vi "CRYXY Graph InsDel.vi"(10 "Graph VI Ref":refnum<vi>, 11 "sAction":string) -> ()   [LabVIEW 2013]
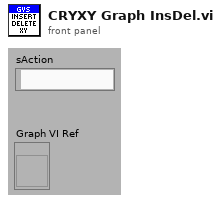
[diagram p1: front panel]
types:
  T1 = typedef "LVBoundsTypeDef.ctl" = cluster{"Width":u32, "Height":u32}
  T2 = enum16{"No Scaling", "Scale All Objects", "Scale Single Object"}
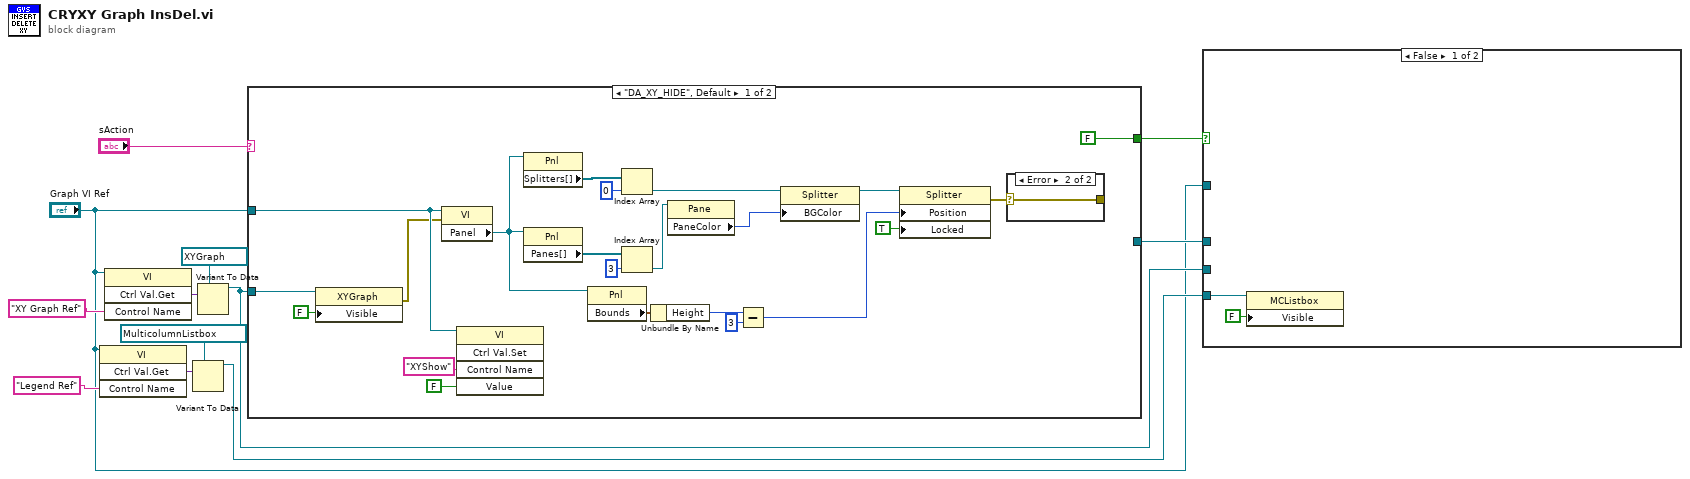
[diagram p0: block diagram]
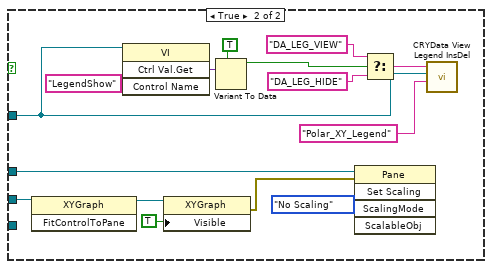
[diagram p2: hidden frame]
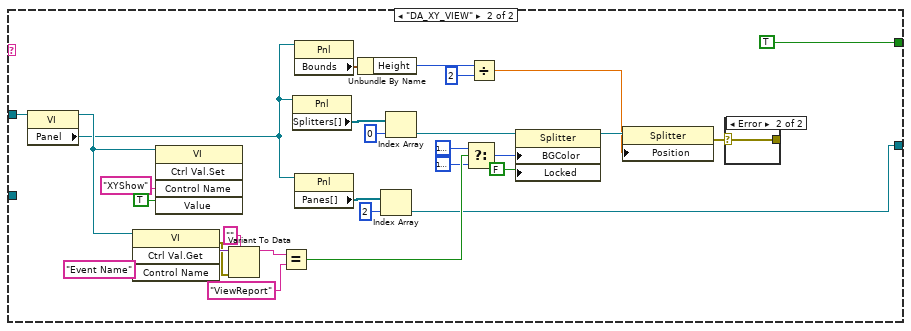
[diagram p4: hidden frame]
diagram:
  n1 = invoke class="VI" method="Ctrl Val.Get"(reference="Graph VI Ref", "Control Name"="Legend Ref") -> ("Get Control Value Variant"=w6:variant)  [unwired: 2 in, 3 out]
  n2 = invoke class="VI" method="Ctrl Val.Get"(reference="Graph VI Ref", "Control Name"="XY Graph Ref") -> ("Get Control Value Variant"=w11:variant)  [unwired: 2 in, 3 out]
  n3 = Variant To Data(type=refnum<vi> refnum ("Legend Ref"), Variant=w6) -> (data=w4:refnum<vi>)  [unwired: 1 in, 1 out]
  n4 = Variant To Data(type=refnum<vi> refnum ("Legend Ref"), Variant=w11) -> (data=w8:refnum<vi>)  [unwired: 1 in, 1 out]
  n5 = case shown="\"DA_XY_HIDE\", Default" "sAction" {
    tunnel: "Graph VI Ref" -> [w34 w63]
    tunnel: w8 -> [w24 _]
    tunnel: [FALSE TRUE] -> w2
    tunnel: [_ w42] -> w3
    frame "DA_XY_HIDE", Default {
      n6 = property class="XYGraph"(reference=w24, "Visible"=FALSE) -> (error out=w16:errorcluster)  [unwired: 1 in, 1 out]
      n7 = property class="VI"(reference=w34, error in=w16) -> ("Panel"=w18:refnum<vi>)  [unwired: 2 out]
      n8 = invoke class="VI" method="Ctrl Val.Set"(reference=w34, "Control Name"="XYShow", "Value"=FALSE ("Visible")) -> ()  [unwired: 2 in, 5 out]
      n9 = property class="Pnl"(reference=w18) -> ("Splitters[]"=w30:refnum<vi>[])  [unwired: 1 in, 2 out]
      n10 = property class="Pnl"(reference=w18) -> ("Panes[]"=w29:refnum<vi>[])  [unwired: 1 in, 2 out]
      n11 = property class="Pnl"(reference=w18) -> ("Bounds"=w21:T1)  [unwired: 1 in, 2 out]
      n12 = Index Array(array=w30, index=0) -> (element=w27:refnum<vi>)
      n13 = Index Array(array=w29, index=3) -> (element=w13:refnum<vi>)
      n14 = Unbundle By Name(w21) -> ("Height"=w20:u32)
      n15 = property class="Pane"(reference=w13) -> ("PaneColor"=w28:u32)  [unwired: 1 in, 2 out]
      n16 = Subtract(x=w20, y=u32 3) -> (x-y=w17:u32)
      n17 = property on="Property Node" class="Splitter"(reference=w27, "BGColor"=w28) -> (reference out=w31:refnum<vi>)  [unwired: 1 in, 1 out]
      n18 = property on="Property Node" class="Splitter"(reference=w31, "Position"=w17, "Locked"=TRUE ("Splitter Position Locked")) -> (error out=w32:errorcluster)  [unwired: 1 in, 1 out]
      n19 = case shown="Error" w32 {
        selector: w32 -> [w35 w36]
        tunnel: [w35 w36] -> _
        frame No Error {
        }
        frame Error {
        }
      }
    }
    frame "DA_XY_VIEW" {
      n20 = property class="VI"(reference=w63) -> (reference out=w53:refnum<vi>, "Panel"=w41:refnum<vi>)  [unwired: 1 in, 1 out]
      n21 = invoke class="VI" method="Ctrl Val.Get"(reference=w53, "Control Name"="Event Name") -> (error out=w56:errorcluster, "Get Control Value Variant"=w57:variant)  [unwired: 2 in, 2 out]
      n22 = invoke class="VI" method="Ctrl Val.Set"(reference=w53, "Control Name"="XYShow", "Value"=TRUE ("Visible")) -> ()  [unwired: 2 in, 5 out]
      n23 = Variant To Data(error in=w56, type="" ("Control Name"), Variant=w57) -> (data=w58:string)  [unwired: 1 out]
      n24 = Equal?(x=w58, y="ViewReport" ("Control Name")) -> (x = y?=w50:bool)
      n25 = property class="Pnl"(reference=w41) -> ("Splitters[]"=w65:refnum<vi>[])  [unwired: 1 in, 2 out]
      n26 = property class="Pnl"(reference=w41) -> ("Bounds"=w64:T1)  [unwired: 1 in, 2 out]
      n27 = property class="Pnl"(reference=w41) -> ("Panes[]"=w43:refnum<vi>[])  [unwired: 1 in, 2 out]
      n28 = Unbundle By Name(w64) -> ("Height"=w47:u32)
      n29 = Index Array(array=w43, index=2) -> (element=w42:refnum<vi>)
      n30 = Index Array(array=w65, index=0) -> (element=w62:refnum<vi>)
      n31 = Select(t=u32 16777226, s=w50, f=u32 16777238) -> (s? t:f=w51:u32)
      n32 = Divide(x=w47, y=u32 2) -> (x/y=w37:dbl)
      n33 = property on="Property Node" class="Splitter"(reference=w62, "BGColor"=w51, "Locked"=FALSE ("Splitter Position Locked")) -> (reference out=w38:refnum<vi>)  [unwired: 1 in, 1 out]
      n34 = property on="Property Node" class="Splitter"(reference=w38, "Position"=w37) -> (error out=w39:errorcluster)  [unwired: 1 in, 1 out]
      n35 = case shown="Error" w39 {
        selector: w39 -> [w66 w67]
        tunnel: [w66 w67] -> _
        frame No Error {
        }
        frame Error {
        }
      }
    }
  }
  n36 = case shown="False" w2 {
    tunnel: w8 -> [_ w84]
    tunnel: w4 -> [w69 _]
    tunnel: w3 -> [_ w80]
    tunnel: "Graph VI Ref" -> [_ w70]
    frame False {
      n37 = property class="MCListbox"(reference=w69, "Visible"=FALSE) -> ()  [unwired: 1 in, 2 out]
    }
    frame True {
      n38 = invoke class="XYGraph" method="FitControlToPane"(reference=w84) -> (reference out=w82:refnum<vi>)  [unwired: 2 in, 2 out]
      n39 = invoke class="VI" method="Ctrl Val.Get"(reference=w70, "Control Name"="LegendShow") -> ("Get Control Value Variant"=w77:variant)  [unwired: 2 in, 3 out]
      n40 = property class="XYGraph"(reference=w82, "Visible"=TRUE) -> (error out=w79:errorcluster)  [unwired: 1 in, 1 out]
      n41 = Variant To Data(type=TRUE, Variant=w77) -> (data=w75:bool)  [unwired: 1 in, 1 out]
      n42 = invoke class="Pane" method="Set Scaling"(reference=w80, error in=w79, "ScalingMode"=T2."No Scaling" ("Scaling Mode")) -> ()  [unwired: 2 in, 5 out]
      n43 = Select(t="DA_LEG_VIEW" ("Action Type"), s=w75, f="DA_LEG_HIDE" ("Action Type")) -> (s? t:f=w72:string)
      n44 = call "CRYData View Legend InsDel.vi"("sOption"="Polar_XY_Legend", "Graph VI Ref"=w70, "sAction"=w72) -> ()  [unwired: 1 in, 8 out]
    }
  }
